vi "Gain Lookup Table.vi"() -> (2 "ROUT<3:0>":u8[](array[numeric])=[15, 14, 13, 12, 11, 10, 9, 8, 0, 1, 2, 3, 4, 5, 6, 7], 3 "Gain(dB)":dbl[](array[numeric])=[1.4, 1.2, 1.0, 0.8, 0.6, 0.4, 0.2, 0.0, -0.2, -0.4, -0.6, -0.8, -1.0, -1.2, -1.4, -1.6])   [LabVIEW 2020]
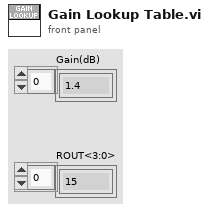
[diagram p1: front panel]
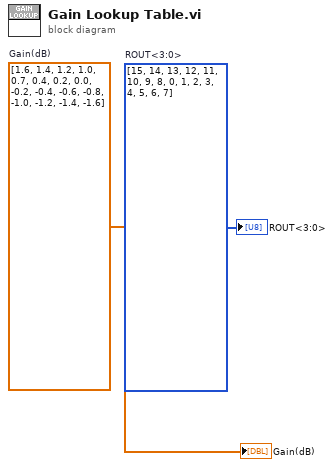
[diagram p0: block diagram]
diagram:
  w1 = u8[] [15, 14, 13, 12, 11, 10, 9, 8, 0, 1, 2, 3, 4, 5, 6, 7]  # ROUT<3:0>
  w2 = dbl[] [1.6, 1.4, 1.2, 1.0, 0.7, 0.4, 0.2, 0.0, -0.2, -0.4, -0.6, -0.8, -1.0, -1.2, -1.4, -1.6]  # Gain(dB)
  "Gain(dB)" <- w2
  "ROUT<3:0>" <- w1
